vi "Vision 차선 최초인식점 2개 좌표변환.vi"(1 "Vision":dbl[][](array[numeric]), 2 "GPS":dbl[][](array[numeric]), 3 "d_vision (GPS와 Vision 사이거리)_측정해서 나중에 상수로 바꾸기":dbl) -> (0 "Lane":dbl[][](array[numeric]))   [LabVIEW 2016]
uses:
  <vilib>/imath/engines/lvmath2/RunTimeEngine/IndexRead/NIMS M(S).vi
  <instcachedir>/0/NIMS M(S)_B826C018497E4940AE96BD27B540B6FB.lvgen/NIMS M(S)_B826C018497E4940AE96BD27B540B6FB_000.vi
  <vilib>/imathl/engines/lvmath/Functions/Error Handling/Create Error.vi
  <vilib>/imath/engines/lvmath2/RunTimeEngine/BuiltInFunctions/deg_to_rad/NIMS_deg_to_rad.vi
  <instcachedir>/0/NIMS_deg_to_rad_4A81D684CE8D4DD79924F5AB74D756E1.lvgen/NIMS_deg_to_rad_4A81D684CE8D4DD79924F5AB74D756E1_001.vi
  <vilib>/imath/engines/lvmath2/RunTimeEngine/IndexRead/NIMS M(S,S).vi
  <instcachedir>/0/NIMS M(S,S)_AC51E74150A542F7991B9634C66F3096.lvgen/NIMS M(S,S)_AC51E74150A542F7991B9634C66F3096_000.vi
  <vilib>/imath/engines/lvmath2/RunTimeEngine/NodeEndStatement/NIMS_NodeEndStatement_Output.vi
  <instcachedir>/0/NIMS_NodeEndStatement_Output_53EC0D466D134D7ABD903AC30B43404B.lvgen/NIMS_NodeEndStatement_Output_53EC0D466D134D7ABD903AC30B43404B_002.vi
  <vilib>/imath/engines/lvmath2/RunTimeEngine/ErrorHandling/NIMS_Finalize Error.vi
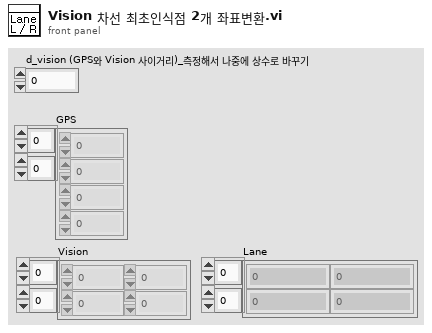
[diagram p1: front panel]
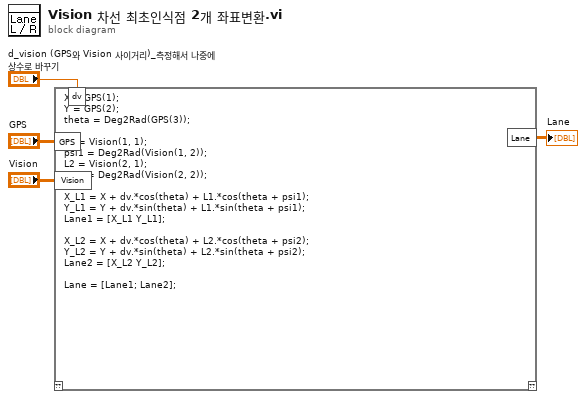
[diagram p0: block diagram]
diagram:
  n1 = mathscript code="X = GPS(1);\nY = GPS(2);\ntheta = Deg2Rad(GPS(3));\n\nL1 = Vision(1, 1);\npsi1 = Deg2Rad(Vision(1, 2));\nL2 = Vision(2, 1);\npsi2 = Deg2Rad(Vision(2, 2));\n\nX_L1 = X + dv.*cos(theta) + L1.*cos(theta + psi1);\nY_L1 = Y + dv.*sin(theta) + L1.*sin(theta + psi1);\nLane1 = [X_L1 Y_L1];\n\nX_L2 = X + dv.*cos(theta) + L2.*cos(theta + psi2);\nY_L2 = Y + dv.*sin(theta) + L2.*sin(theta + psi2);\nLane2 = [X_L2 Y_L2];\n\nLane = [Lane1; Lane2];"("GPS"="GPS", "dv"="d_vision (GPS와 Vision 사이거리)_측정해서 나중에 상수로 바꾸기", "Vision"="Vision") -> ("Lane"=→"Lane":dbl[][])  [unwired: 1 in, 1 out]
